vi "Nico's PID controler.vi"(4 "PID gains":T6={"proportional gain (Kc)"=1.0, "integral time (Ti, min)"=0.01, "derivative time (Td, min)"=0.0} {"derivative time (Td, min)" format="%.3f"; "integral time (Ti, min)" format="%.3f"; "proportional gain (Kc)" format="%#.6g"}, 5 "error in":errorcluster, 6 "Reversed?":bool, 7 "Speed to acheive":dbl, 8 "MotorControlDeviceRef":T1) -> (3 "MotorControlDeviceRef 2":T1)   [LabVIEW 2018]
uses:
  <vilib>/Rock Robotics/WPI/MotorControl/WPI_MotorControlDeviceRef.ctl
  <vilib>/Rock Robotics/WPI/MotorControl/WPI_MotorControlType.ctl
  <vilib>/Rock Robotics/SystemInterfaces/DIO/FPGA_DIOPWMChannel.ctl
  <vilib>/Rock Robotics/WPI/PWM/WPI_PWMDeadband.ctl
  <vilib>/Rock Robotics/SystemInterfaces/DIO/FPGA_DIOChannel.ctl
  <vilib>/Rock Robotics/WPI/ThirdParty/REV Robotics/SPARK MAX/Typedef/Spark MAX Control Type.ctl
  <vilib>/addons/control/pid/pid.llb/PID (DBL).vi
  <vilib>/addons/control/pid/NI_PID_pid.lvlib
  <vilib>/ptbypt/NI_PtbyPt.lvlib
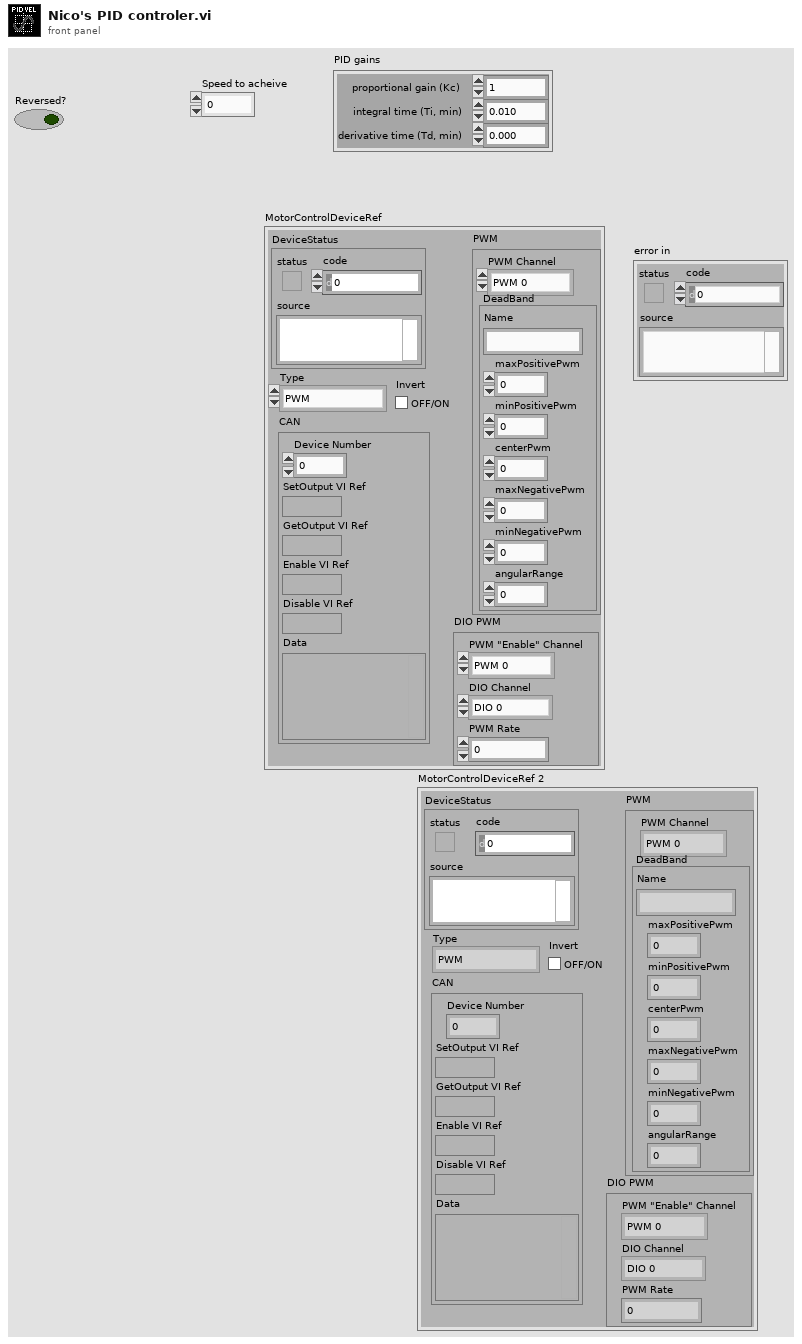
[diagram p1: front panel]
types:
  T1 = typedef "WPI_MotorControlDeviceRef.ctl" = cluster{"DeviceStatus":errorcluster, "Type":T2, "PWM":cluster{"PWM Channel":T3, "DeadBand":T4}, "CAN":cluster{"Device Number":u8, "SetOutput VI Ref":variant, "GetOutput VI Ref":variant, "Enable VI Ref":variant, "Disable VI Ref":variant, "Data":variant}, "Invert":bool, "DIO PWM":cluster{"PWM \"Enable\" Channel":T3, "DIOChannel":T5, "PWM Rate":dbl}}
  T2 = typedef "WPI_MotorControlType.ctl" = enum16{"PWM", "CAN", "DIO PWM"}
  T3 = typedef "FPGA_DIOPWMChannel.ctl" = enum8{"PWM 0", "PWM 1", "PWM 2", "PWM 3", "PWM 4", "PWM 5", "PWM 6", "PWM 7", "PWM 8", "PWM 9", "PWM MXP 0", "PWM MXP 1", "PWM MXP 2", "PWM MXP 3", "PWM MXP 4", "PWM MXP 5", "PWM MXP 6", "PWM MXP 7", "PWM MXP 8", "PWM MXP 9", "Invalid"}
  T4 = typedef "WPI_PWMDeadband.ctl" = cluster{"Name":string, "maxPositivePwm":i32, "minPositivePwm":i32, "centerPwm":i32, "maxNegativePwm":i32, "minNegativePwm":i32, "angularRange":u16}
  T5 = typedef "FPGA_DIOChannel.ctl" = enum8{"DIO 0", "DIO 1", "DIO 2", "DIO 3", "DIO 4", "DIO 5", "DIO 6", "DIO 7", "DIO 8", "DIO 9", "DIO MXP 0", "DIO MXP 1", "DIO MXP 2", "DIO MXP 3", "DIO MXP 4", "DIO MXP 5", "DIO MXP 6", "DIO MXP 7", "DIO MXP 8", "DIO MXP 9", "DIO MXP 10", "DIO MXP 11", "DIO MXP 12", "DIO MXP 13", "DIO MXP 14", "DIO MXP 15", "SPI Port CS1", "SPI Port CS2", "SPI Port CS3", "SPI Port MISO", "SPI Port MOSI", "Invalid"}
  T6 = cluster{"proportional gain (Kc)":dbl, "integral time (Ti, min)":dbl, "derivative time (Td, min)":dbl}
  T7 = typedef "Spark MAX Control Type.ctl" = enum16{"Percent VBus", "Voltage", "Velocity", "Position"}
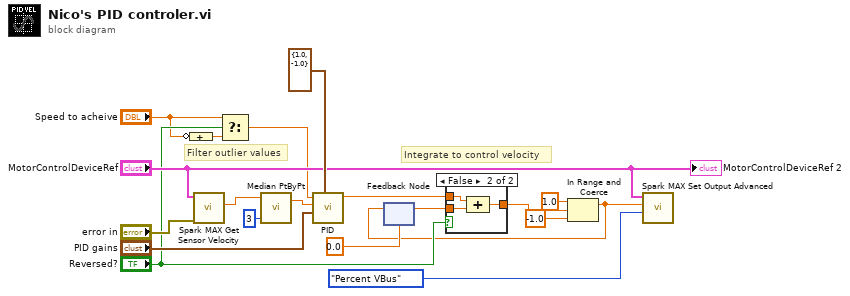
[diagram p0: block diagram]
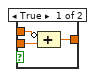
[diagram p2: hidden frame]
diagram:
  # "Integrate to control velocity"
  # "Filter outlier values"
  n1 = Compound Arithmetic op=ADD(invert "Speed to acheive") -> (w6:dbl)
  n2 = call <vilib>:"Spark MAX Get Sensor Velocity.vi"("error in (no error)"="error in", "MotorControlDevRef in"="MotorControlDeviceRef") -> ("Sensor Velocity"=w9:dbl)  [unwired: 6 in, 3 out]
  n3 = Select(t="Speed to acheive", s="Reversed?", f=w6) -> (s? t:f=w5:dbl)
  n4 = call <vilib>:"Median PtByPt.vi"("sample length"=3, "x"=w9) -> ("median"=w10:dbl)  [unwired: 2 in, 1 out]
  n5 = call-poly <vilib>:"PID.vi"("output range"=cluster{"output high":dbl, "output low":dbl} {"output high"=1.0, "output low"=-1.0}, "PID gains"="PID gains", "process variable"=w10, "setpoint"=w5) -> ("output"=w14:dbl)  [unwired: 6 in, 1 out]
  n6 = feedback #1(0.0) -> (w13:dbl)
  n7 = case shown="False" "Reversed?" {
    tunnel: w14 -> [w22 w25]
    tunnel: w13 -> [w21 w24]
    tunnel: [w20 w23] -> w4
    frame True {
      n8 = Compound Arithmetic op=ADD(invert w22, w21) -> (w20:dbl)
    }
    frame False {
      n9 = Compound Arithmetic op=ADD(w25, w24) -> (w23:dbl)
    }
  }
  n10 = In Range and Coerce(upper limit=1.0, x=w4, lower limit=-1.0) -> (coerced(x)=w3:dbl)  [unwired: 1 out]
  n11 = feedback-in #1(w3) -> ()
  n12 = call <vilib>:"Spark MAX Set Output Advanced.vi"("Control Mode"=Spark_MAX_Control_Type."Percent VBus", "Setpoint"=w3, "MotorControlDevRef"="MotorControlDeviceRef") -> ()  [unwired: 7 in, 2 out]
  "MotorControlDeviceRef 2" <- "MotorControlDeviceRef"
